vi "RSZVB Set Sweep Single - All Chans.vi"(8 "error in (no error)":errorcluster {"code" format="%.0x"}, 10 "Single Sweep (1: Continuous Sweep)":i32(ring)=1 items=["Single Channel", "All Channels"], 11 "VISA session":refnum<visa-resource-name>) -> (0 "error out":errorcluster {"code" format="%.0x"}, 3 "dup VISA session":refnum<visa-resource-name>)   [LabVIEW 2011]
doc: "This function selects the scope of the single sweep sequence.\n\nNote(s):\n\n(1) The setting is applied in single sweep mode only.\n\nRemote-control command(s):\nINITiate<Ch>[:IMMediate]:SCOPe ALL | SINGle"
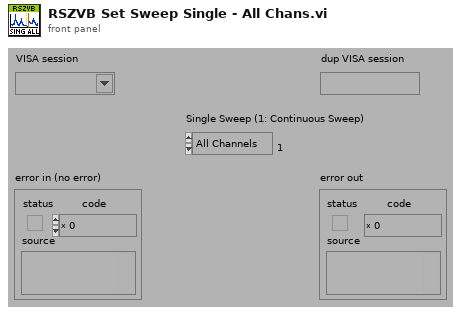
[diagram p1: front panel]
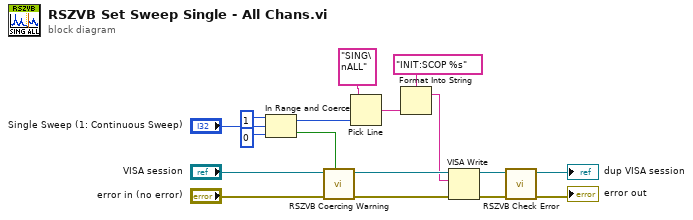
[diagram p0: block diagram]
diagram:
  n1 = In Range and Coerce(upper limit=1, x="Single Sweep (1: Continuous Sweep)", lower limit=0) -> (coerced(x)=w14:i32, In Range?=w8:bool)
  n2 = call "RSZVB Coercing Warning.vi"("In Range?"=w8, "error in (no error)"="error in (no error)", "VISA session"="VISA session") -> ("error out"=w11:errorcluster, "dup VISA session"=w12:refnum<visa-resource-name>)  [unwired: 7 in]
  n3 = Pick Line(multi-line string="SING\nALL", line index=w14) -> (output string=w1:string)  [unwired: 1 in]
  n4 = Format Into String(format string="INIT:SCOP %s", w1) -> (resulting string=w7:string)  [unwired: 2 in, 1 out]
  n5 = VISA Write(VISA resource name=w12, write buffer=w7, error in (no error)=w11) -> (VISA resource name out=w9:refnum<visa-resource-name>, error out=w10:errorcluster)  [unwired: 1 out]
  n6 = call "RSZVB Check Error.vi"("error in (no error)"=w10, "VISA session"=w9) -> ("error out"=→"error out":errorcluster, "dup VISA session"=→"dup VISA session":refnum<visa-resource-name>)  [unwired: 8 in]
